vi "listbox.vi"() -> ()   [LabVIEW 2018]
doc: "Demonstrates the use of the Listbox control."
panel:
  in  "Stop":bool
  out "Multiple Selections":string[](array[string])
  out "Multiple Selection Listbox Value":i32[](array[numeric])
  in  "Multiple Selection Listbox":i32[](listbox)=[0, 2, 4]
  out "Single Selection":string
  out "Single Selection Listbox Value":i32
  in  "Single Selection Listbox":i32(listbox)
  # "Based on LabVIEW Example (Help -> Find Examples...)"
  # "Overview: Demonstrates the use of the Listbox control.\nInstructions:\n1. Select an item in the Single Selection Listbox.\n2. Select multiple items in the Multiple Selection Listbox by Ctrl-clicking the items (or Cmd-clicking on Mac OS).\n3. Run the VI. The values and names of the selected items are displayed."
  # "To change the listbox selection mode, right-click on the listbox and change the Selection Mode."
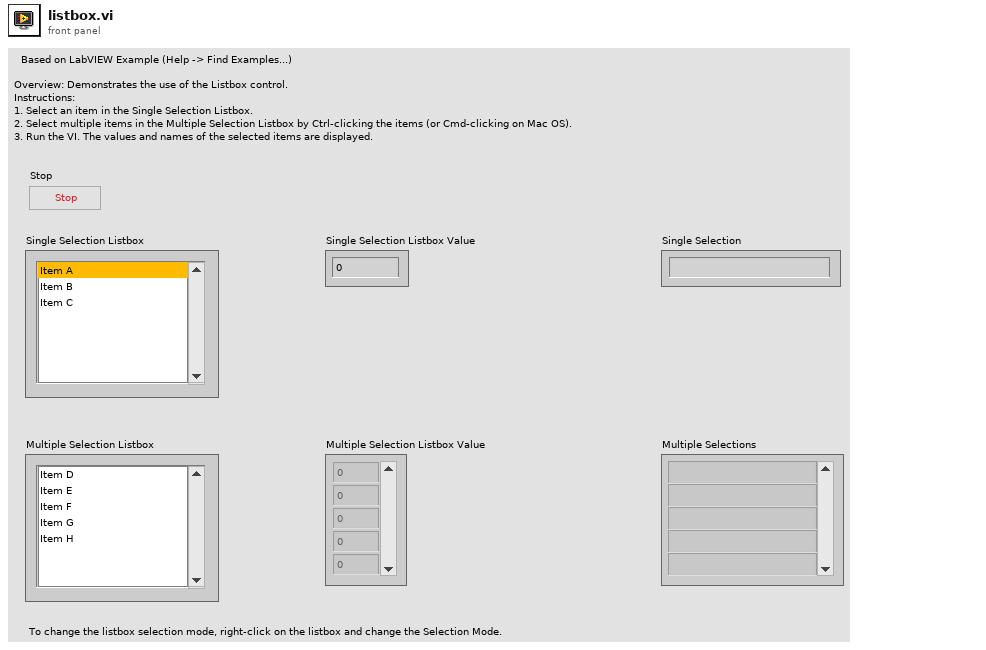
[diagram p1: front panel]
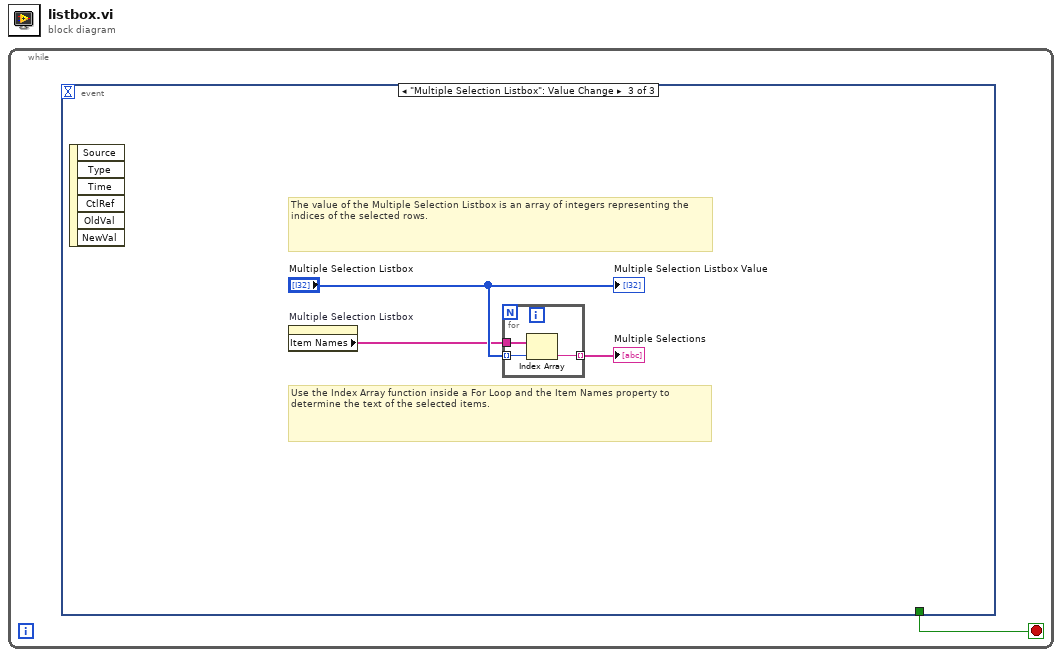
[diagram p0: block diagram]
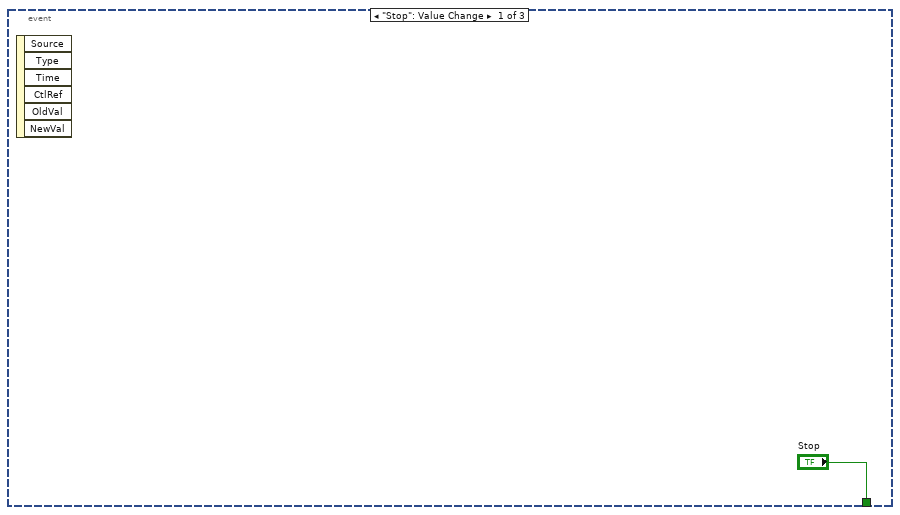
[diagram p2: hidden frame]
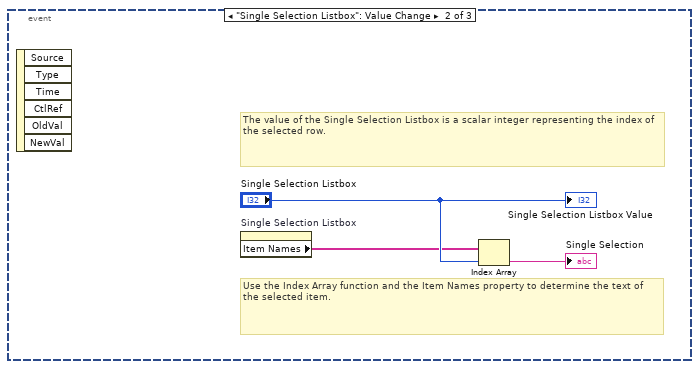
[diagram p3: hidden frame]
diagram:
  n1 = while {
    stop <- w1 stop-if-true
    n2 = event shown="[2] \"Multiple Selection Listbox\": Value Change" {
      selector: _ -> [_ _ _]
      dyn-events: _ -> [_ _ _]
      timeout: _ -> [_ _ _]
      tunnel: ["Stop" _ _] -> w1
      event "Stop": Value Change {
        n3 = event-data() -> ()  [unwired: 1 in, 6 out]
      }
      event "Single Selection Listbox": Value Change {
        # "Use the Index Array function and the Item Names property to determine the text of the selected item."
        # "The value of the Single Selection Listbox is a scalar integer representing the index of the selected row."
        n4 = event-data() -> ()  [unwired: 1 in, 6 out]
        n5 = property on="Single Selection Listbox" class="ListBox (strict)"() -> ("Item Names"=w3:string[])  [unwired: 2 in, 2 out]
        n6 = Index Array(array=w3, index="Single Selection Listbox") -> (element=→"Single Selection":string)
        "Single Selection Listbox Value" <- "Single Selection Listbox"
      }
      event "Multiple Selection Listbox": Value Change {
        # "Use the Index Array function inside a For Loop and the Item Names property to determine the text of the selected items."
        # "The value of the Multiple Selection Listbox is an array of integers representing the indices of the selected rows."
        n7 = event-data() -> ()  [unwired: 1 in, 6 out]
        n8 = property on="Multiple Selection Listbox" class="LstBox (strict)"() -> ("Item Names"=w6:string[])  [unwired: 2 in, 2 out]
        n9 = for {
          tunnel: w6 -> [w11]
          tunnel: "Multiple Selection Listbox" -> [w10] mode=indexing
          tunnel: [w9] -> w8 mode=indexing
          n10 = Index Array(array=w11, index=w10) -> (element=w9:string)
        }
        "Multiple Selections" <- w8
        "Multiple Selection Listbox Value" <- "Multiple Selection Listbox"
      }
    }
  }
